vi "DI ADC Address.vi"(10 "DI ADC Select":T2, 11 "DCM - RT in":refnum<class "DCM - RT.lvclass">) -> (2 "DI ADC Addresses":T1 {"DI ADC 4" format="%.0x"; "DI ADC 3" format="%.0x"; "DI ADC 2" format="%.0x"; "DI ADC 1" format="%.0x"}, 3 "DCM - RT out":refnum<class "DCM - RT.lvclass">)   [LabVIEW 2016, in "DCM-Classes.lvlib" / "DCM - RT.lvclass"]
uses:
  DCM - RT.lvclass
  DI - ADC Select.ctl
  <vilib>/Powertrain Controls/Device Drivers/DCM/Rev0/FPGA/DI - ADC Signals.ctl
  <vilib>/Powertrain Controls/Device Drivers/DCM/Rev0/FPGA/DI - ADC Address.ctl
  <vilib>/Powertrain Controls/Device Drivers/DCM/Rev0/FPGA/DCM - FPGA.lvlib
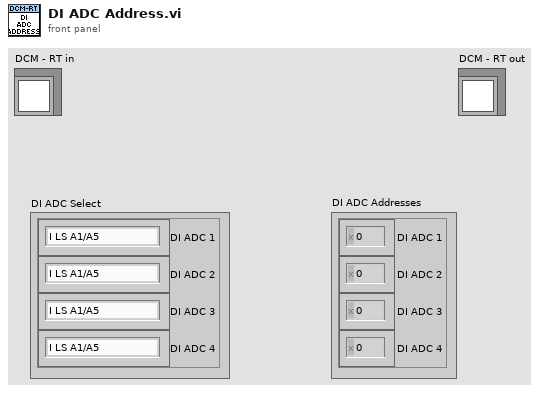
[diagram p1: front panel]
types:
  T1 = typedef "DCM - FPGA.lvlib/DI - ADC Address.ctl" = cluster{"DI ADC 1":u8, "DI ADC 2":u8, "DI ADC 3":u8, "DI ADC 4":u8}
  T2 = typedef "DCM-Classes.lvlib/DCM - RT.lvclass/DI - ADC Select.ctl" = cluster{"DI ADC 1":T3, "DI ADC 2":T3, "DI ADC 3":T3, "DI ADC 4":T3}
  T3 = typedef "DCM - FPGA.lvlib/DI - ADC Signals.ctl" = enum8{"I LS A1/A5", "I LS A2/A6", "I LS A3/A7", "I LS A4", "I LS A8/PumpA", "V PZ A1", "V PZ A2", "V PZ A3", "V PZ A4", "V S A1", "V S A2", "V S A3", "V S A4", "V S A5", "V S A6", "V S A7", "V S A8", "V Pump A", "V Secondary A1A2", "V Secondary A3A4", "V Ext HV A", "------------------------ ", "I LS B1/B5", "I LS B2/B6", "I LS B3/B7", "I LS B4", "I LS B8/PumpB", "V PZ B1", "V PZ B2", "V PZ B3", "V PZ B4", "V S B1", "V S B2", "V S B3", "V S B4", "V S B5", "V S B6", "V S B7", "V S B8", "V Pump B", "V Secondary B1B2", "V Secondary B3B4", "V Ext HV B", "-------------------------  ", "AI 1", "AI 2", "AI 3", "AI 4", "AI 5", "AI 6", "AI 7", "AI 8", "AI 9", "AI 10", "AI 11", "AI 12", "-------------------------   ", "V DRVP"}
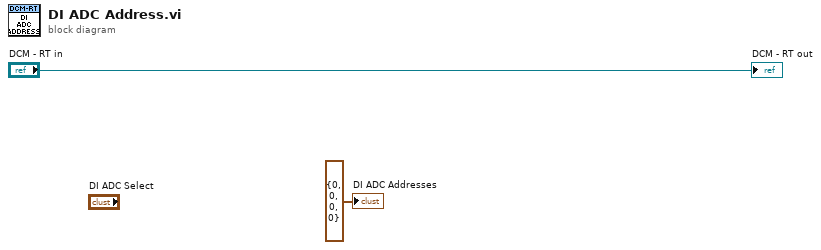
[diagram p0: block diagram]
diagram:
  "DCM - RT out" <- "DCM - RT in"
  "DI ADC Addresses" <- T1 {"DI ADC 1"=0, "DI ADC 2"=0, "DI ADC 3"=0, "DI ADC 4"=0} ("DI ADC Addresses")
